vi "read.vi"(11 "input string":string="(+ hello (/ 2 3 4))") -> (3 "Expression out":T1)   [LabVIEW 2020]
uses:
  ExpressionType.ctl
  Expression.ctl
panel:
  out "Tokens 2":string[](array[string])
  out "Tokens":string[](array[string])
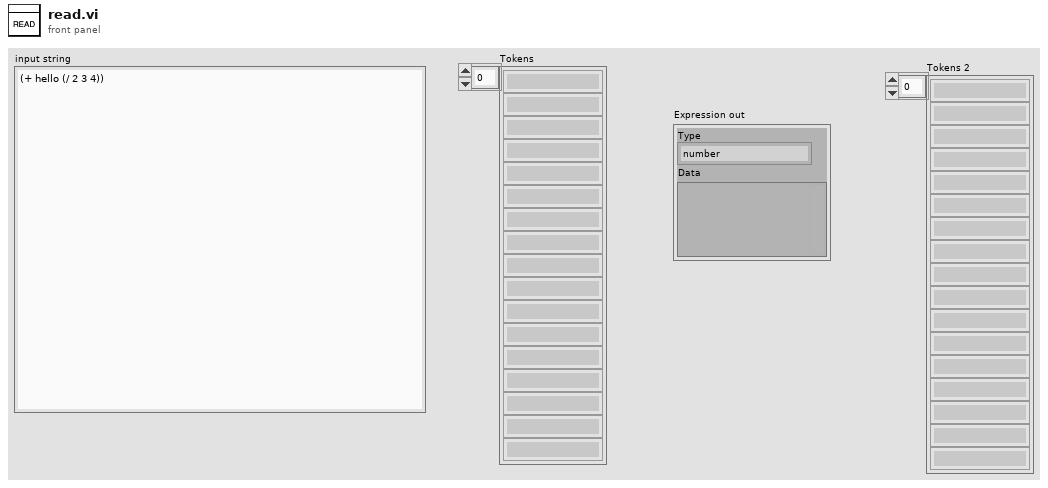
[diagram p1: front panel]
types:
  T1 = typedef "Expression.ctl" = cluster{"Type":T2, "Data":variant}
  T2 = typedef "ExpressionType.ctl" = enum16{"number", "string", "symbol", "primitive", "list", "closure", "macro", "nil", "error"}
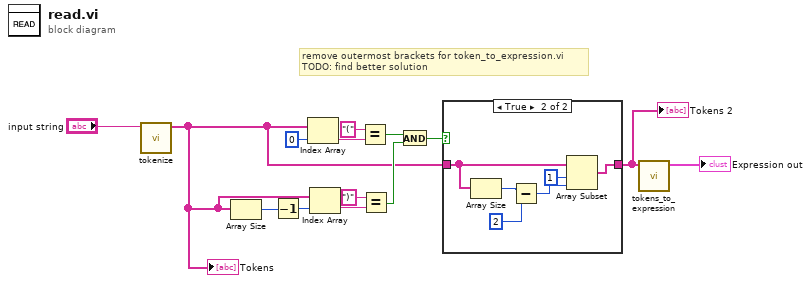
[diagram p0: block diagram]
diagram:
  # "remove outermost brackets for token_to_expression.vi\nTODO: find better solution"
  n1 = call "tokenize.vi"("input string"="input string") -> ("Tokens"=w2:string[])  [unwired: 10 in]
  "Tokens" <- w2
  n2 = Array Size(array=w2) -> (size(s)=w11:i32)
  n3 = Decrement(x=w11) -> (x-1=w10:i32)
  n4 = Index Array(array=w2, index=0) -> (element=w9:string)
  n5 = Index Array(array=w2, index=w10) -> (element=w6:string)
  n6 = Equal?(x="(", y=w9) -> (x = y?=w4:bool)
  n7 = Equal?(x=")", y=w6) -> (x = y?=w5:bool)
  n8 = And(x=w4, y=w5) -> (x .and. y?=w3:bool)
  n9 = case shown="True" w3 {
    tunnel: w2 -> [w15 w20]
    tunnel: [w15 w19] -> w1
    frame False {
    }
    frame True {
      n10 = Array Size(array=w20) -> (size(s)=w18:i32)
      n11 = Subtract(x=w18, y=2) -> (x-y=w17:i32)
      n12 = Array Subset(array=w20, index=1, length=w17) -> (w19:string[])
    }
  }
  "Tokens 2" <- w1
  n13 = call "tokens_to_expression.vi"("Tokens in"=w1) -> ("Expression out"=→"Expression out":T1)  [unwired: 9 in, 1 out]
